vi "Main.vi"() -> ()   [LabVIEW 2018]
doc: "This template is for the Queued Message Handler design pattern.\n\nThe Event Handling Loop generates messages based on user interface actions.\n\nThe Message Handling Loop processes messages generated by the Event Handling Loop, or by other messages. The messages are string values, so new messages can be added easily to the Message Cases case structure in the Message Handling Loop. Each message cluster can also provide an optional value for Message Data, which is a variant that can be converted to whatever message-specific data is required."
uses:
  Snake/Type Defs/Coordinates.ctl
  Snake/Type Defs/Direction.ctl
  Game Board/Game Board.lvclass/Game Board.ctl
  Game Board/Generate.vi
  Snake/Output Snake Coordinates.vi
  Game Board/Replace Board Pixel.vi
  Snake/Snake.lvclass
  Game Board/Game Board.lvclass
  Fruit/Fruit.lvclass
panel:
  out "Score":u32
  out "Board":u32[][](array[colorbox])
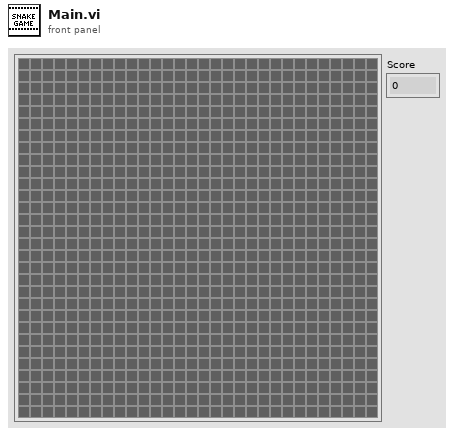
[diagram p1: front panel]
types:
  T1 = typedef "Coordinates.ctl" = cluster{"X":i32, "Y":i32}
  T2 = typedef "Direction.ctl" = enum16{"Up", "Down", "Left", "Right"}
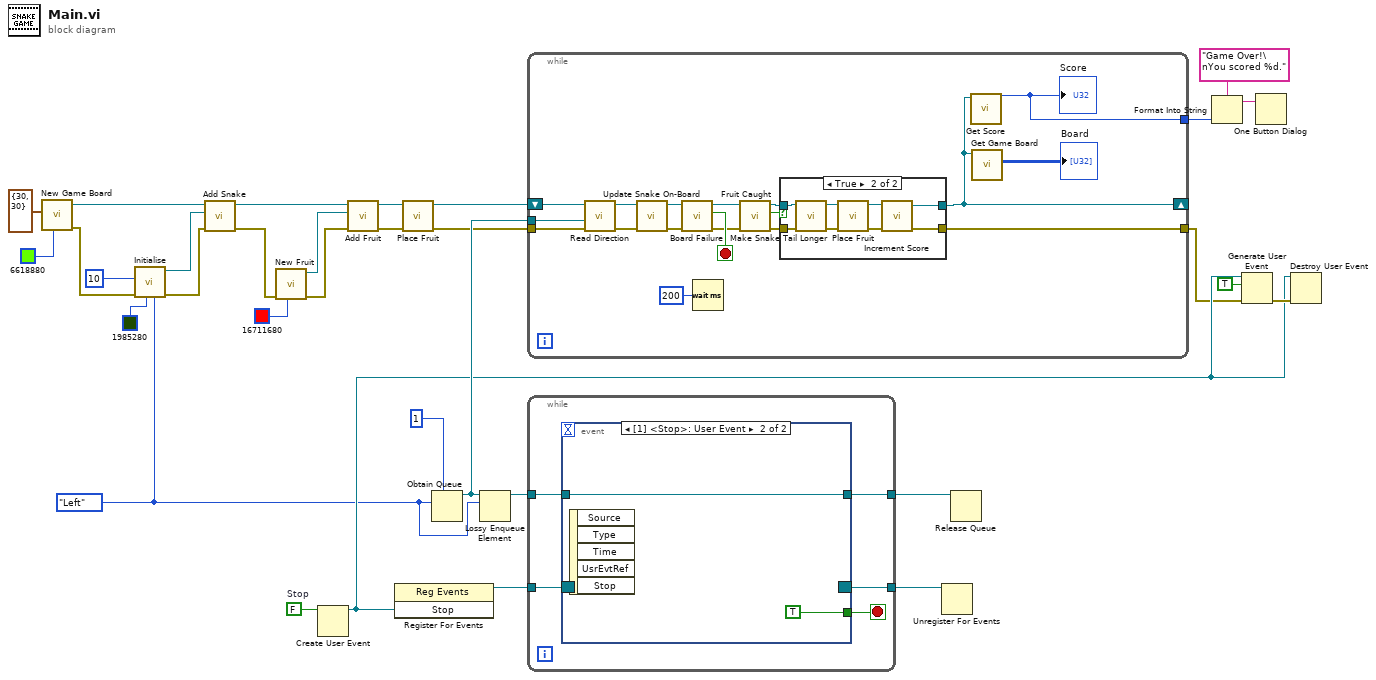
[diagram p0: block diagram]
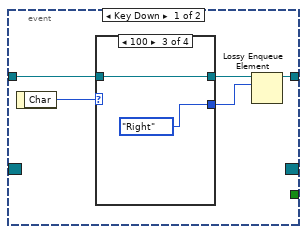
[diagram p2: hidden frame]
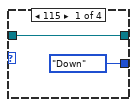
[diagram p3: hidden frame]
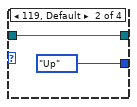
[diagram p4: hidden frame]
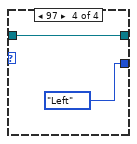
[diagram p5: hidden frame]
diagram:
  w26 = FALSE  # Stop
  w18 = Direction."Left" ("Direction")
  n1 = call "New Game Board.vi"("Color Box"=u32 6618880, "Grid Size"=T1 {"X"=30, "Y"=30}) -> ("error out"=w10:errorcluster, "Game Board out"=w17:refnum<class "Game Board.lvclass">)  [unwired: 8 in]
  n2 = call "Initialise.vi"("Direction"=w18, "Snake Colour"=u32 1985280, "error in (no error)"=w10, "Starting Elements"=10) -> ("error out"=w11:errorcluster, "Snake out"=w16:refnum<class "Snake.lvclass">)  [unwired: 6 in]
  n3 = call "Add Snake.vi"("error in (no error)"=w11, "Snake in"=w16, "Game Board in"=w17) -> ("error out"=w12:errorcluster, "Game Board out"=w13:refnum<class "Game Board.lvclass">)  [unwired: 7 in]
  n4 = call "New Fruit.vi"("Color Box"=u32 16711680, "error in (no error)"=w12) -> ("error out"=w9:errorcluster, "Fruit out"=w14:refnum<class "Fruit.lvclass">)  [unwired: 8 in]
  n5 = Create User Event(user event datatype=w26) -> (user event=w23:refnum<user-event>)  [unwired: 1 in, 1 out]
  n6 = call "Add Fruit.vi"("error in (no error)"=w9, "Fruit.lvclass"=w14, "Game Board in"=w13) -> ("error out"=w7:errorcluster, "Game Board out"=w8:refnum<class "Game Board.lvclass">)  [unwired: 7 in]
  n7 = register-events(w23) -> (reference out=w28:refnum<event-registration>)  [unwired: 2 in, 1 out]
  n8 = call "Place Fruit.vi"("error in (no error)"=w7, "Game Board in"=w8) -> ("error out"=w5:errorcluster, "Game Board out"=w6:refnum<class "Game Board.lvclass">)  [unwired: 8 in]
  n9 = Obtain Queue(max queue size (-1, unlimited)=1, element data type=w18) -> (queue out=w29:refnum<queue>)  [unwired: 3 in, 2 out]
  n10 = Lossy Enqueue Element(queue=w29, element=w18) -> (queue out=w30:refnum<queue>)  [unwired: 1 in, 3 out]
  n11 = while {
    tunnel: w29 -> [w48]
    tunnel: w5 -> [w47]
    shift-right: [w35] -> _
    shift-left: w6 -> [w49]
    tunnel: [w36] -> w4
    tunnel: [w33] -> w3
    stop <- w41 stop-if-true
    n12 = call "Read Direction.vi"("error in (no error)"=w47, "Direction SEQ"=w48, "Game Board in"=w49) -> ("error out"=w45:errorcluster, "Game Board out"=w46:refnum<class "Game Board.lvclass">)  [unwired: 7 in]
    n13 = call "Update Snake On-Board.vi"("error in (no error)"=w45, "Game Board in"=w46) -> ("error out"=w42:errorcluster, "Game Board out"=w43:refnum<class "Game Board.lvclass">)  [unwired: 8 in]
    n14 = call "Board Failure.vi"("error in (no error)"=w42, "Game Board in"=w43) -> ("error out"=w39:errorcluster, "Fail"=w41:bool, "Game Board out"=w40:refnum<class "Game Board.lvclass">)  [unwired: 7 in]
    n15 = Wait (ms)(milliseconds to wait=u32 200) -> ()  [unwired: 1 out]
    n16 = call "Fruit Caught.vi"("error in (no error)"=w39, "Game Board in"=w40) -> ("error out"=w37:errorcluster, "Fruit Caught"=w34:bool, "Game Board out"=w38:refnum<class "Game Board.lvclass">)  [unwired: 7 in]
    n17 = case shown="True" w34 {
      tunnel: w38 -> [w52 w60]
      tunnel: w37 -> [w51 w59]
      tunnel: [w52 w54] -> w35
      tunnel: [w51 w53] -> w36
      frame False {
      }
      frame True {
        n18 = call "Make Snake Tail Longer.vi"("error in (no error)"=w59, "Game Board in"=w60) -> ("error out"=w57:errorcluster, "Game Board out"=w58:refnum<class "Game Board.lvclass">)  [unwired: 8 in]
        n19 = call "Place Fruit.vi"("error in (no error)"=w57, "Game Board in"=w58) -> ("error out"=w55:errorcluster, "Game Board out"=w56:refnum<class "Game Board.lvclass">)  [unwired: 8 in]
        n20 = call "Increment Score.vi"("error in (no error)"=w55, "Game Board in"=w56) -> ("error out"=w53:errorcluster, "Game Board out"=w54:refnum<class "Game Board.lvclass">)  [unwired: 8 in]
      }
    }
    n21 = call "Get Score.vi"("Game Board in"=w35) -> ("Score"=w33:u32)  [unwired: 10 in]
    "Score" <- w33
    n22 = call "Get Game Board.vi"("Game Board in"=w35) -> ("Game Board"=→"Board":u32[][])  [unwired: 10 in]
  }
  n23 = while {
    tunnel: w30 -> [w65]
    tunnel: [w64] -> w31
    tunnel: w28 -> [w63]
    tunnel: [w62] -> w27
    stop <- w61 stop-if-true
    n24 = event shown="[1] <Stop>: User Event" {
      selector: w63 -> [_ _]
      dyn-events: [_ _] -> w62
      timeout: _ -> [_ _]
      tunnel: w65 -> [w69 w79]
      tunnel: [w66 w79] -> w64
      tunnel: [_ TRUE] -> w61
      event Key Down {
        n25 = event-data() -> ("Char"=w70:i16)  [unwired: 1 in]
        n26 = case shown="100" w70 {
          tunnel: w69 -> [w72 w74 w76 w78]
          tunnel: [w72 w74 w76 w78] -> w68
          tunnel: [Direction."Down" ("Direction") Direction."Up" ("Direction") Direction."Right" ("Direction") Direction."Left" ("Direction")] -> w67
          frame 115 {
          }
          frame 119, Default {
          }
          frame 100 {
          }
          frame 97 {
          }
        }
        n27 = Lossy Enqueue Element(queue=w68, element=w67) -> (queue out=w66:refnum<queue>)  [unwired: 1 in, 3 out]
      }
      event User Event {
        n28 = event-data() -> ()  [unwired: 1 in, 5 out]
      }
    }
  }
  n29 = Unregister For Events(event registration refnum=w27) -> ()  [unwired: 1 in, 1 out]
  n30 = Release Queue(queue=w31) -> ()  [unwired: 2 in, 3 out]
  n31 = Format Into String(format string="Game Over!\nYou scored %d.", w3) -> (resulting string=w2:string)  [unwired: 2 in, 1 out]
  n32 = Generate User Event(user event=w23, event data cluster=TRUE ("event data"), error in=w4) -> (error out=w24:errorcluster)  [unwired: 1 in, 1 out]
  n33 = One Button Dialog(message=w2) -> ()  [unwired: 1 in, 1 out]
  n34 = Destroy User Event(user event=w23, error in=w24) -> ()  [unwired: 1 out]
